vi "Launch.vi"() -> ()   [LabVIEW 2021, in "TemplatePlugin.lvlib"]
uses:
  TemplatePlugin.lvlib
  Class/TemplatePlugin.lvclass
  C:/Program Files/National Instruments/LabVIEW 2021/vi.lib/CIF Foundation/CIF Core/CIFCore/Class/CIFCorePlugin.lvclass
  <vilib>/CIF Foundation/CIF Core/CIFCore/Class/CIFCorePlugin.lvclass/CIFCorePlugin.ctl
  <vilib>/CIF Foundation/CIF Core/CIFCore/Class/CIFCorePlugin.lvclass
  <vilib>/CIF Foundation/CIF Core/CIFUtilities/CIFLogs/CIFLogs.lvlib
panel:
  out "error out":errorcluster
  out "gRPC Server Port":i32
  in  "Plugin Name":string="template"
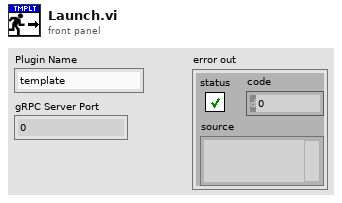
[diagram p1: front panel]
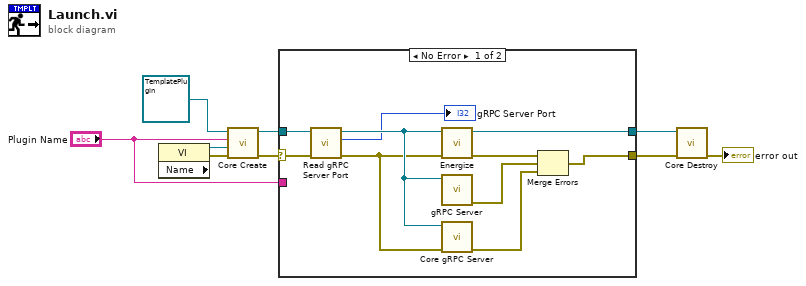
[diagram p0: block diagram]
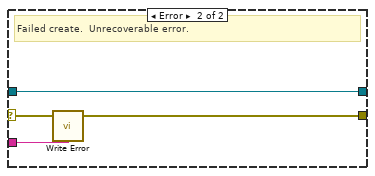
[diagram p2: hidden frame]
diagram:
  n1 = property class="VI" props=["Name"]() -> (reference out=w7:refnum<vi>, error out=w8:errorcluster)  [unwired: 2 in, 1 out]
  n2 = call <vilib>:"Core Create.vi"("error in (no error)"=w8, "VI Reference"=w7, "Plugin Name"="Plugin Name", "CIFTemplateNode in"=refnum<class "TemplatePlugin.lvclass"> refnum ("CIFTemplatePlugin.lvclass")) -> ("error out"=w5:errorcluster, "CIFTemplateNode out"=w4:refnum<class "TemplatePlugin.lvclass">)  [unwired: 6 in]
  n3 = case shown="No Error" w5 {
    selector: w5 -> [w14 w21]
    tunnel: [w19 w22] -> w9
    tunnel: w4 -> [w18 w22]
    tunnel: [w16 w20] -> w2
    tunnel: "Plugin Name" -> [_ w23]
    frame No Error {
      n4 = call <vilib>:"Read gRPC Server Port.vi"("error in (no error)"=w14, "CIFTemplateNode in"=w18) -> ("error out"=w13:errorcluster, "gRPC Server Port"=→"gRPC Server Port":i32, "CIFTemplateNode out"=w15:refnum<class "TemplatePlugin.lvclass">)  [unwired: 7 in]
      n5 = call "Energize.vi"("error in (no error)"=w13, "CIFTemplatePlugin in"=w15) -> ("error out"=w17:errorcluster, "CIFTemplatePlugin out"=w19:refnum<class "TemplatePlugin.lvclass">)  [unwired: 8 in]
      n6 = call "gRPC Server.vi"("CIFTemplatePlugin in"=w15) -> ("error out"=w12:errorcluster)  [unwired: 9 in, 1 out]
      n7 = call <vilib>:"Core gRPC Server.vi"("error in (no error)"=w13, "CIFTemplateNode in"=w15) -> ("error out"=w11:errorcluster)  [unwired: 8 in, 1 out]
      n8 = Merge Errors(w17, w12, w11) -> (w16:errorcluster)
    }
    frame Error {
      # "Failed create.  Unrecoverable error."
      n9 = call <vilib>:"Write Error.vi"("error in (no error)"=w21, "Plugin Name"=w23) -> ("cleared error"=w20:errorcluster)  [unwired: 2 in]
    }
  }
  n10 = call <vilib>:"Core Destroy.vi"("error in (no error)"=w2, "CIFTemplateNode in"=w9) -> ("error out"=→"error out":errorcluster)  [unwired: 8 in, 1 out]
